vi "Socket_test.vi"() -> ()   [LabVIEW 2019]
panel:
  in  "stop":bool
  out "data out":string
  # "Labview server"
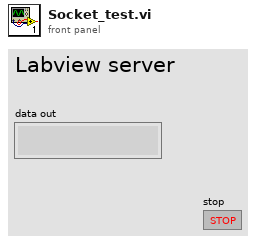
[diagram p1: front panel]
types:
  T1 = enum16{"Standard", "Buffered", "CRLF", "Immediate"}
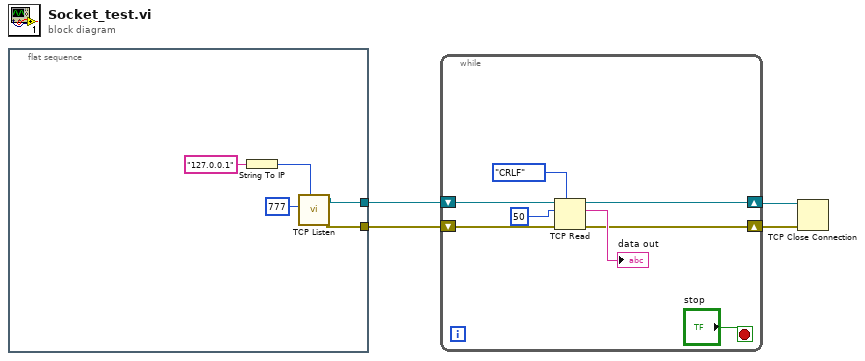
[diagram p0: block diagram]
diagram:
  n1 = flat-sequence {
    tunnel: [w9] -> w4
    tunnel: [w8] -> w1
    frame #0 {
      n2 = String To IP(1:"127.0.0.1" ("name")) -> (0:w5:u32)
      n3 = call <vilib>:"TCP Listen.vi"("net address"=w5, "port"=u16 777) -> ("error out"=w8:errorcluster, "connection ID"=w9:refnum<k5>)  [unwired: 5 in, 3 out]
    }
  }
  n4 = while {
    shift-right: [w17] -> w3
    shift-left: w4 -> [w16]
    shift-right: [w13] -> w2
    shift-left: w1 -> [w12]
    stop <- "stop" stop-if-true
    n5 = TCP Read(connection ID=w16, bytes to read=50 ("timeout ms (25000)"), error in (no error)=w12, 7:T1."CRLF" ("mode (standard)")) -> (connection ID out=w17:refnum<k5>, data out=→"data out":string, error out=w13:errorcluster)  [unwired: 1 in]
  }
  n6 = TCP Close Connection(connection ID=w3, error in (no error)=w2) -> ()  [unwired: 1 in, 2 out]
